vi "array_median_double.vi"(1 "Input Array":dbl[](array[numeric])) -> (0 "Median":dbl)   [LabVIEW 2019]
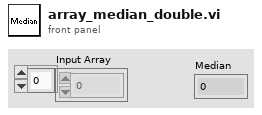
[diagram p1: front panel]
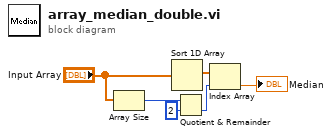
[diagram p0: block diagram]
diagram:
  n1 = Array Size(array="Input Array") -> (size(s)=w2:i32)
  n2 = Sort 1D Array(array="Input Array") -> (sorted array=w6:dbl[])
  n3 = Quotient & Remainder(x=w2, y=2) -> (floor(x/y)=w4:i32)  [unwired: 1 out]
  n4 = Index Array(array=w6, index=w4) -> (element=→"Median":dbl)
